vi "Tool_Unicode Update Table Headers.vi"(6 "Caption":string, 7 "Interpret as Unicode (T)":bool=TRUE, 8 "error in (no error)":errorcluster, 9 "Row Headers[]":string[](array[string]), 10 "Column Headers[]":string[](array[string]), 11 "Table Ref":refnum<vi>) -> (0 "error out":errorcluster, 3 "Table Ref":refnum<vi>)   [LabVIEW 2009]
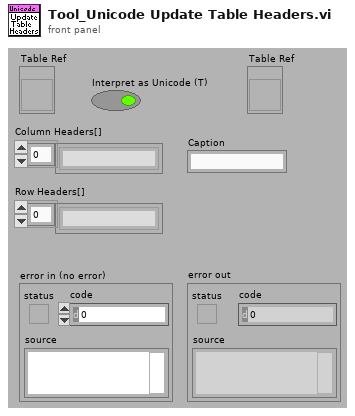
[diagram p1: front panel]
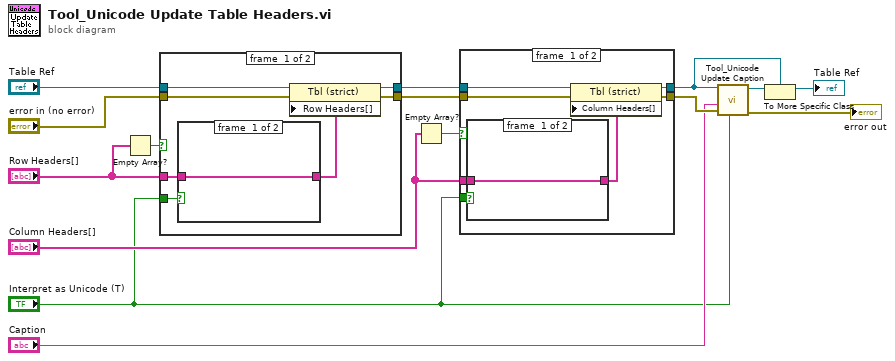
[diagram p0: block diagram]
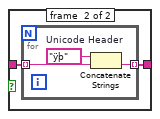
[diagram p2: hidden frame]
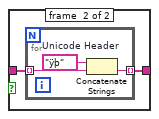
[diagram p4: hidden frame]
diagram:
  n1 = Empty Array?(array="Row Headers[]") -> (empty?=w12:bool)
  n2 = case shown="False" w12 {
    tunnel: "Row Headers[]" -> [w22 _]
    tunnel: "Table Ref" -> [w20 w30]
    tunnel: "error in (no error)" -> [w19 w29]
    tunnel: [w18 w30] -> w13
    tunnel: "Interpret as Unicode (T)" -> [w17 _]
    tunnel: [w16 w29] -> w8
    frame #0 {
      n3 = case shown="False" w17 {
        tunnel: w22 -> [w23 w25]
        tunnel: [w23 w24] -> w21
        frame #0 {
        }
        frame #1 {
          n4 = for {
            tunnel: w25 -> [w28] mode=indexing
            tunnel: [w27] -> w24 mode=indexing
            w26 = "ÿþ"  # Unicode Header
            n5 = Concatenate Strings(w26, w28) -> (w27:string)
          }
        }
      }
      n6 = property class="Tbl (strict)"(reference=w20, error in=w19, "Row Headers[]"=w21) -> (reference out=w18:refnum<vi>, error out=w16:errorcluster)
    }
    frame #1 {
    }
  }
  n7 = Empty Array?(array="Column Headers[]") -> (empty?=w9:bool)
  n8 = case shown="False" w9 {
    tunnel: "Column Headers[]" -> [w37 _]
    tunnel: [w36 w45] -> w7
    tunnel: w8 -> [w34 w45]
    tunnel: w13 -> [w33 w44]
    tunnel: "Interpret as Unicode (T)" -> [w32 _]
    tunnel: [w31 w44] -> w4
    frame #0 {
      n9 = case shown="False" w32 {
        tunnel: w37 -> [w38 w40]
        tunnel: [w38 w39] -> w35
        frame #0 {
        }
        frame #1 {
          n10 = for {
            tunnel: w40 -> [w43] mode=indexing
            tunnel: [w42] -> w39 mode=indexing
            w41 = "ÿþ"  # Unicode Header
            n11 = Concatenate Strings(w41, w43) -> (w42:string)
          }
        }
      }
      n12 = property class="Tbl (strict)"(reference=w33, error in=w34, "Column Headers[]"=w35) -> (reference out=w31:refnum<vi>, error out=w36:errorcluster)
    }
    frame #1 {
    }
  }
  n13 = call "Tool_Unicode Update Caption.vi"("Interpret as Unicode (T)"="Interpret as Unicode (T)", "error in (no error)"=w7, "Caption"="Caption", "Control Reference"=w4) -> ("error out"=→"error out":errorcluster, "Control Reference"=w5:refnum<vi>)  [unwired: 4 in]
  n14 = To More Specific Class(target class=w4, reference=w5) -> (specific class reference=→"Table Ref":refnum<vi>)  [unwired: 1 in, 1 out]
